vi "Validate Existing Connections.vi"(8 "error in":errorcluster, 10 "validation information in":T1={"Missing Modules"=variant(cluster{"ID":string, "Path":string}[] []), "Module Connection Map"=variant, "Unused Modules"=variant(cluster{"ID":string, "Path":string}[] [])}, 11 "routing and faulting in":T2 format="%.0x") -> (0 "error out":errorcluster, 1 "connection errors":errorcluster[](array[cluster]), 2 "validation information out":T1, 3 "routing and faulting out":T2 format="%.0x")   [LabVIEW 2020, in "Routing and Faulting Scripting.lvlib"]
uses:
  Routing and Faulting Scripting.lvlib
  <vilib>/NI VeriStand/Custom Device API/Custom Device Item Ref.ctl
  Validation Information.ctl
  Routing Channel/Routing Channel Error Information.ctl
  <vilib>/NI VeriStand/Custom Device API/Custom Device API.lvlib
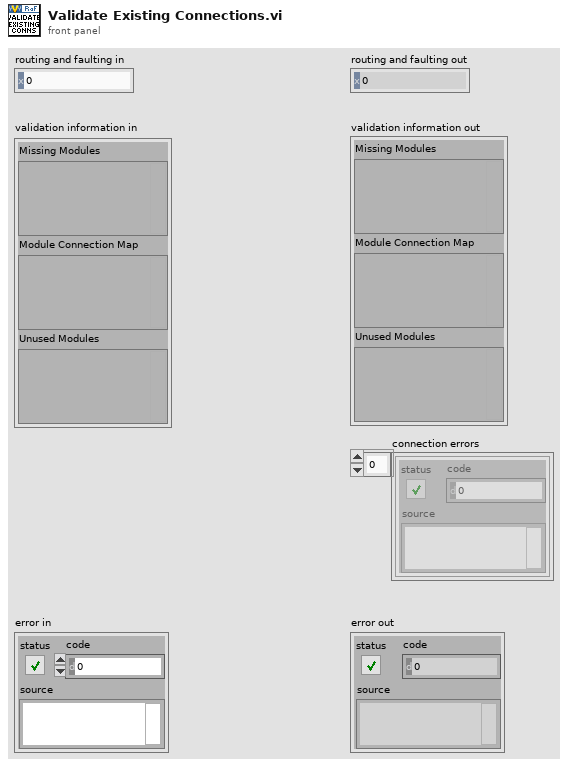
[diagram p1: front panel]
types:
  T1 = typedef "Routing and Faulting Scripting.lvlib/Validation Information.ctl" = cluster{"Missing Modules":variant, "Module Connection Map":variant, "Unused Modules":variant}
  T2 = typedef "Custom Device API.lvlib/Custom Device Item Ref.ctl" = u64
  T3 = typedef "Routing and Faulting Scripting.lvlib/Routing Channel Error Information.ctl" = cluster{"Channel Name":string, "State":string, "Module":string}
  T4 = typedef "Routing and Faulting Shared.lvlib/Channel States.ctl" = T5[]
  T5 = typedef "Routing and Faulting Shared.lvlib/Routing State.ctl" = cluster{"Name":string, "Description":string, "Value":i32, "Connection List":T6[]}
  T6 = typedef "Routing and Faulting Shared.lvlib/Connection.ctl" = cluster{"Module":string, "Source":string, "Destination":string}
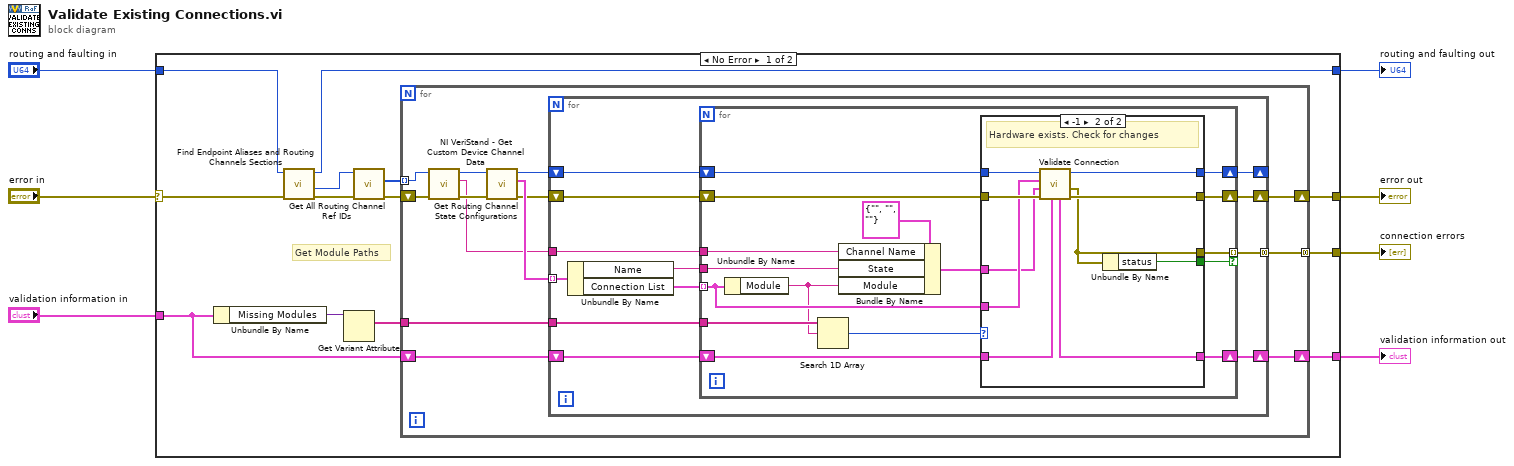
[diagram p0: block diagram]
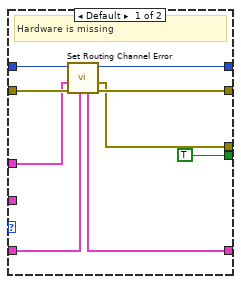
[diagram p2: hidden frame]
diagram:
  n1 = case shown="No Error" "error in" {
    selector: "error in" -> [w20 w83]
    tunnel: "routing and faulting in" -> [w9 w82]
    tunnel: [w17 w83] -> w5
    tunnel: [w19 w82] -> w4
    tunnel: [w13 _] -> w3
    tunnel: "validation information in" -> [w10 w81]
    tunnel: [w8 w81] -> w1
    frame No Error {
      # "Get Module Paths"
      n2 = Unbundle By Name(w10) -> ("Missing Modules"=w11:variant)
      n3 = call "Find Endpoint Aliases and Routing Channels Sections.vi"("error in"=w20, "routing and faulting custom device in"=w9) -> ("error out"=w16:errorcluster, "routing channels"=w18:T2, "routing and faulting custom device out"=w19:T2)  [unwired: 6 in, 1 out]
      n4 = Get Variant Attribute(Variant=w11) -> (names=w12:string[])  [unwired: 3 in, 3 out]
      n5 = call "Get All Routing Channel Ref IDs.vi"("error in"=w16, "routing channels in"=w18) -> ("error out"=w15:errorcluster, "all routing channels"=w14:T2[])  [unwired: 7 in, 1 out]
      n6 = for {
        tunnel: w14 -> [w27] mode=indexing
        shift-right: [w29] -> w17
        shift-left: w15 -> [w28]
        tunnel: w12 -> [w32]
        tunnel: [w24] -> w13 mode=concatenating
        shift-right: [w21] -> w8
        shift-left: w10 -> [w22]
        n7 = call <vilib>:"NI VeriStand - Get Custom Device Channel Data.vi"("error in (no error)"=w28, "Channel Ref in"=w27) -> ("error out"=w25:errorcluster, "Channel Name"=w23:string, "Channel Ref out"=w26:T2)  [unwired: 4 in, 3 out]
        n8 = call "Get Routing Channel State Configurations.vi"("error in"=w25, "routing channel in"=w26) -> ("error out"=w31:errorcluster, "state configurations"=w33:T4, "routing channel out"=w30:T2)  [unwired: 7 in]
        n9 = for {
          tunnel: w33 -> [w44] mode=indexing
          tunnel: w32 -> [w43]
          shift-right: [w40] -> w29
          shift-left: w31 -> [w42]
          shift-right: [w39] -> _
          shift-left: w30 -> [w41]
          tunnel: [w37] -> w24 mode=concatenating
          tunnel: w23 -> [w36]
          shift-right: [w34] -> w21
          shift-left: w22 -> [w35]
          n10 = Unbundle By Name(w44) -> ("Name"=w38:string, "Connection List"=w45:T6[])
          n11 = for {
            tunnel: w45 -> [w51] mode=indexing
            tunnel: w43 -> [w61]
            shift-right: [w57] -> w40
            shift-left: w42 -> [w59]
            shift-right: [w56] -> w39
            shift-left: w41 -> [w58]
            tunnel: [w55] -> w37 mode=indexing if=w54
            tunnel: w38 -> [w48]
            tunnel: w36 -> [w49]
            shift-right: [w52] -> w34
            shift-left: w35 -> [w53]
            n12 = Unbundle By Name(w51) -> ("Module"=w47:string)
            n13 = Search 1D Array(1D array=w61, element=w47) -> (index of element=w60:i32)  [unwired: 1 in]
            n14 = Bundle By Name(cluster=T3 {"Channel Name"="", "State"="", "Module"=""} ("Routing Channel Error Information"), "Channel Name"=w49, "State"=w48, "Module"=w47) -> (w46:T3)
            n15 = case shown="-1" w60 {
              tunnel: w59 -> [w69 w80]
              tunnel: w58 -> [w66 w79]
              tunnel: [w68 w77] -> w57
              tunnel: [w67 w76] -> w56
              tunnel: [w65 w75] -> w55
              tunnel: [TRUE w74] -> w54
              tunnel: w53 -> [w63 w72]
              tunnel: [w62 w71] -> w52
              tunnel: w51 -> [_ w78]
              tunnel: w46 -> [w64 w73]
              frame Default {
                # "Hardware is missing"
                n16 = call "Set Routing Channel Error.vi"("validation information in"=w63, "error in"=w69, "routing channel error information"=w64, "routing channel in"=w66) -> ("error out"=w68:errorcluster, "veristand error out"=w65:errorcluster, "routing channel out"=w67:T2, "validation information out"=w62:T1)  [unwired: 4 in]
              }
              frame -1 {
                # "Hardware exists. Check for changes"
                n17 = call "Validate Connection.vi"("validation information in"=w72, "error in"=w80, "routing channel error information"=w73, "connection"=w78, "routing channel in"=w79) -> ("error out"=w77:errorcluster, "veristand error out"=w75:errorcluster, "routing channel out"=w76:T2, "validation information out"=w71:T1)  [unwired: 3 in]
                n18 = Unbundle By Name(w75) -> ("status"=w74:bool)
              }
            }
          }
        }
      }
    }
    frame Error {
    }
  }
  "routing and faulting out" <- w4
  "error out" <- w5
  "connection errors" <- w3
  "validation information out" <- w1
